vi "蠕动泵2动作命令 (子VI).vi"(8 "Error in":errorcluster caption="Error in (no error)", 10 "启动命令":T1(ring), 11 "仪器":enum16{"", "氨氮", "总磷", "总氮", "CODMn", "CODCr"}(ring)=enum."氨氮") -> (0 "error out":errorcluster)   [LabVIEW 2016, in "质控单元.lvlib"]
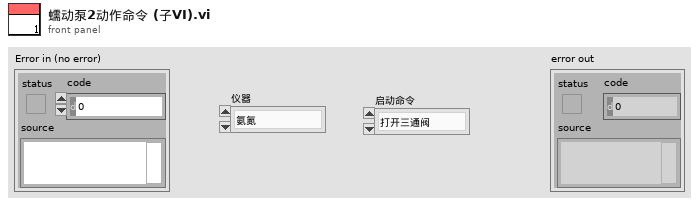
[diagram p1: front panel]
types:
  T1 = enum16{"打开三通阀", "关闭三通阀", "蠕动泵正转", "蠕动泵反转", "蠕动泵停止"}
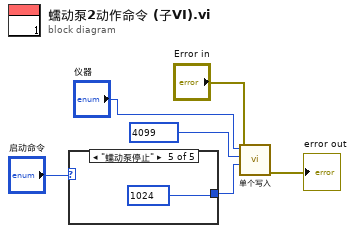
[diagram p0: block diagram]
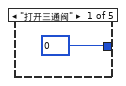
[diagram p2: hidden frame]
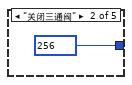
[diagram p3: hidden frame]
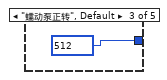
[diagram p4: hidden frame]
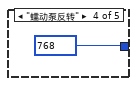
[diagram p5: hidden frame]
diagram:
  n1 = case shown="\"蠕动泵停止\"" "启动命令" {
    tunnel: [u16 0 ("starting address") u16 256 ("starting address") u16 512 ("starting address") u16 768 ("starting address") u16 1024 ("starting address")] -> w2
    frame "打开三通阀" {
    }
    frame "关闭三通阀" {
    }
    frame "蠕动泵正转", Default {
    }
    frame "蠕动泵反转" {
    }
    frame "蠕动泵停止" {
    }
  }
  n2 = call "单个写入.vi"("Error in"="Error in", "value"=w2, "address"=u16 4099 ("starting address"), "Slave ID"="仪器") -> ("error out"=→"error out":errorcluster)  [unwired: 7 in]
